vi "excelReport1.vi"(6 "device":string, 7 "Customer":string, 8 "Shift":string(combo), 9 "End Date":string="2014/9/24", 11 "From Date":string="2014/9/20") -> ()   [LabVIEW 2012]
uses:
  <vilib>/Utility/NIReport.llb/Generate Report Object Reference.ctl
  <vilib>/Utility/NIReport.llb/NI_report.lvclass
  <vilib>/addons/database/Auxilliary.llb/DB Tools Cursor Type.ctl
  <vilib>/addons/database/Connection.llb/DB Tools Open Connec (Path).vi
  <vilib>/addons/database/Connection.llb/Conn Execute.vi
  <vilib>/addons/database/Recordset.llb/Rec Fetch Recordset Data (R).vi
  <vilib>/addons/database/Recordset.llb/Rec Destroy - Connection.vi
  <vilib>/Utility/NIReport.llb/Append Text Table to Report (wrap).vi
  <vilib>/addons/database/_DB Variant To Data/Database Variant To Data.xnode
  <vilib>/addons/database/NI_Database_API.lvlib
  <vilib>/Utility/NIReport.llb/Excel/NI_Excel.lvclass
  <vilib>/addons/_office/NI_ReportGenerationToolkit.lvlib
panel:
  out "Row Headers":string[](array[string])
  out "error out":errorcluster
  out "report out":T1
  in  "Report Template":path=path "c:/m100/data/AT.xls"
  in  "Running":string[][](table)
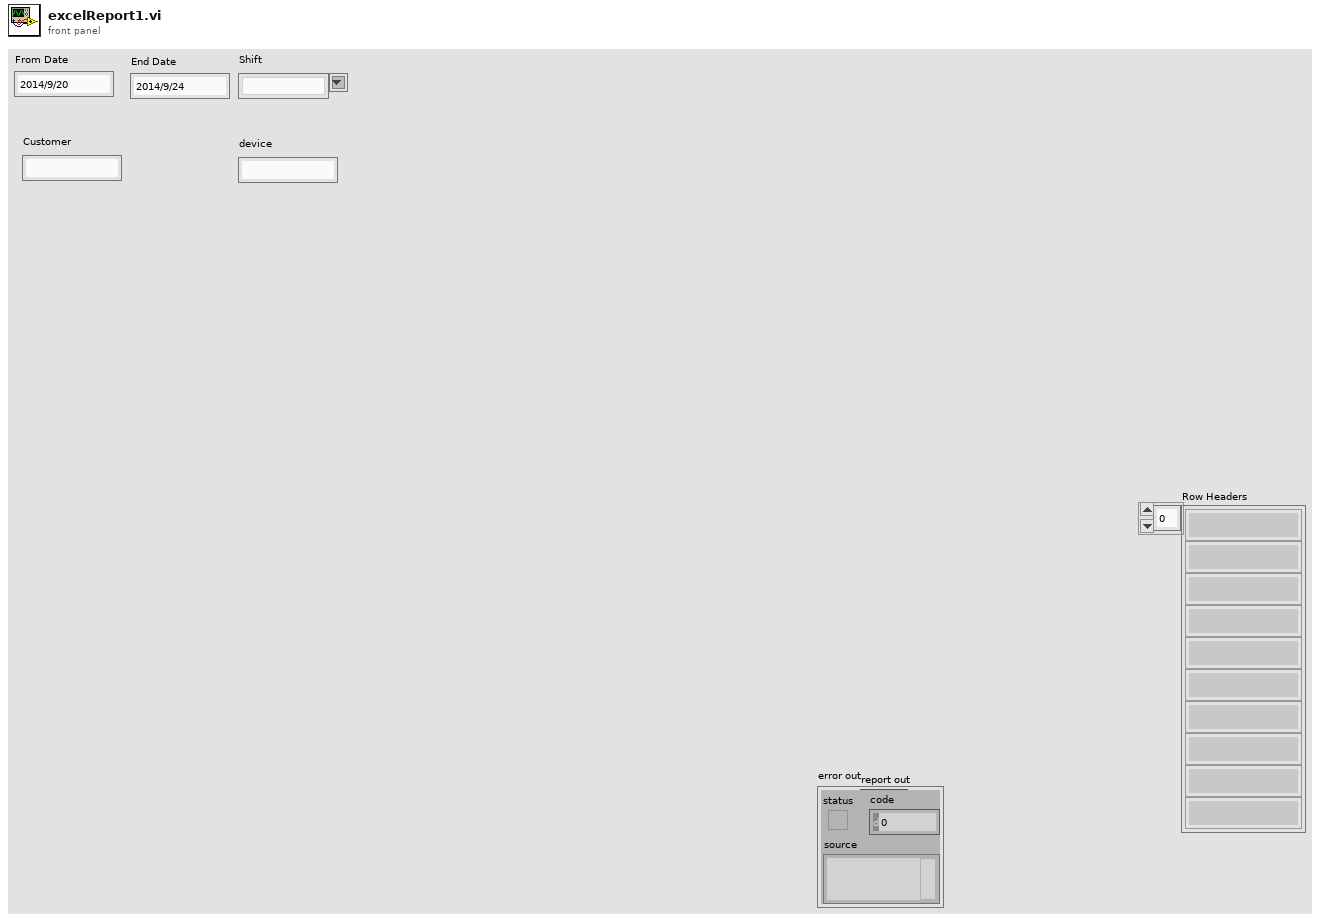
[diagram p1: front panel]
types:
  T1 = typedef "Generate Report Object Reference.ctl" = refnum<class "NI_report.lvclass">
  T2 = typedef "NI_Database_API.lvlib/DB Tools Cursor Type.ctl" = enum16{"forward-only", "keyset", "dynamic", "static"}
  T3 = typedef "NI_Database_API.lvlib/Conn ObjectReference.ctl" = refnum<k1>
  T4 = typedef "NI_Database_API.lvlib/Rec ObjectReference.ctl" = refnum<k1>
  T5 = enum16{"Standard Report", "HTML", "Word", "Excel"}
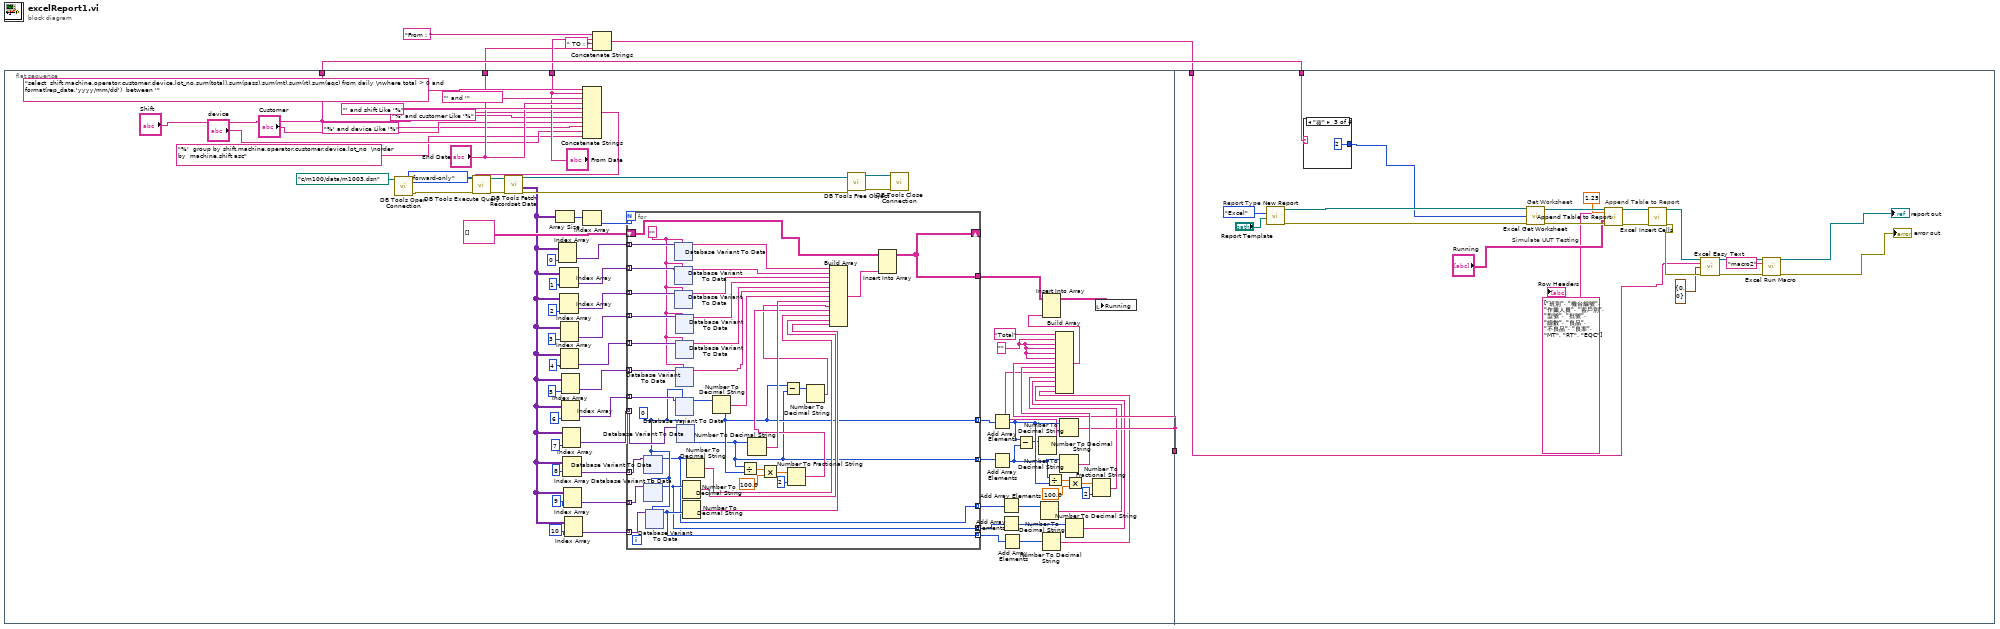
[diagram p0: block diagram]
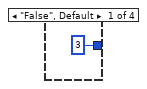
[diagram p2: hidden frame]
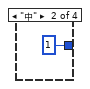
[diagram p3: hidden frame]
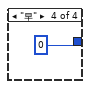
[diagram p4: hidden frame]
diagram:
  n1 = flat-sequence {
    tunnel: [w42] -> w7
    tunnel: ["Shift"] -> w6
    tunnel: ["From Date"] -> w4
    tunnel: ["End Date"] -> w2
    tunnel: w7 -> [_]
    tunnel: w6 -> [w481]
    tunnel: w1 -> [w479]
    frame #0 {
      w57 = "" ("element")
      n2 = call-poly <vilib>:"DB Tools Open Connection.vi"("connection information"=path "c:/m100/data/m1003.dsn") -> ("error out"=w47:errorcluster, "connection reference"=w48:T3)  [unwired: 7 in]
      n3 = Concatenate Strings("select  shift,machine,operator,customer,device,lot_no,sum(total),sum(pass),sum(mt),sum(rt),sum(eqc) from daily \nwhere total > 0 and  format(rep_date,'yyyy/mm/dd')  between '" ("string"), "From Date", "' and '" ("string"), "End Date", "' and shift Like '%" ("string"), "Shift", "%' and customer Like '%" ("string"), "Customer", "%' and device Like '%" ("string"), "device", "%'  group by shift,machine,operator,customer,device,lot_no  \norder by  machine,shift asc" ("string")) -> (w44:string)
      n4 = call-poly <vilib>:"DB Tools Execute Query.vi"("error in (no error)"=w47, "cursor type"=DB_Tools_Cursor_Type."forward-only", "SQL query"=w44, "connection reference"=w48) -> ("error out"=w50:errorcluster, "recordset reference"=w49:T4)  [unwired: 4 in]
      n5 = call-poly <vilib>:"DB Tools Fetch Recordset Data.vi"("error in (no error)"=w50, "recordset reference"=w49) -> ("error out"=w46:errorcluster, "recordset data"=w8:variant[][], "recordset reference out"=w45:T4)  [unwired: 3 in]
      n6 = Array Size(array=w8) -> (size(s)=w81:i32[])
      n7 = Index Array(array=w8, index (col)=0) -> (element=w70:variant[])  [unwired: 1 in]
      n8 = Index Array(array=w8, index (col)=1) -> (element=w77:variant[])  [unwired: 1 in]
      n9 = Index Array(array=w8, index (col)=2) -> (element=w69:variant[])  [unwired: 1 in]
      n10 = Index Array(array=w8, index (col)=3) -> (element=w68:variant[])  [unwired: 1 in]
      n11 = Index Array(array=w8, index (col)=4) -> (element=w67:variant[])  [unwired: 1 in]
      n12 = Index Array(array=w8, index (col)=5) -> (element=w63:variant[])  [unwired: 1 in]
      n13 = Index Array(array=w8, index (col)=6) -> (element=w66:variant[])  [unwired: 1 in]
      n14 = Index Array(array=w8, index (col)=7) -> (element=w65:variant[])  [unwired: 1 in]
      n15 = Index Array(array=w8, index (col)=8) -> (element=w31:variant[])  [unwired: 1 in]
      n16 = Index Array(array=w8, index (col)=9) -> (element=w30:variant[])  [unwired: 1 in]
      n17 = Index Array(array=w8, index (col)=10) -> (element=w29:variant[])  [unwired: 1 in]
      n18 = Index Array(array=w81) -> (element=w80:i32)  [unwired: 1 in]
      n19 = for {
        N: w80 -> [_]
        tunnel: w77 -> [w119] mode=indexing
        tunnel: w65 -> [w121] mode=indexing
        shift-right: [w98] -> _
        shift-left: string[][] [] -> [w105]
        tunnel: w70 -> [w120] mode=indexing
        tunnel: w69 -> [w118] mode=indexing
        tunnel: w68 -> [w117] mode=indexing
        tunnel: w67 -> [w116] mode=indexing
        tunnel: w66 -> [w115] mode=indexing
        tunnel: w63 -> [w112] mode=indexing
        tunnel: [w86] -> w18 mode=indexing
        tunnel: [w85] -> w61 mode=indexing
        tunnel: [w98] -> w40
        tunnel: w31 -> [w97] mode=indexing
        tunnel: w30 -> [w96] mode=indexing
        tunnel: w29 -> [w95] mode=indexing
        tunnel: [w93] -> w26 mode=indexing
        tunnel: [w92] -> w27 mode=indexing
        tunnel: [w91] -> w28 mode=indexing
        w94 = 0
        w111 = ""
        n20 = xnode "Database Variant To Data"("database variant"=w97, "type"=w94) -> ("data"=w91:i32)  [unwired: 1 in, 1 out]
        n21 = xnode "Database Variant To Data"("database variant"=w96, "type"=w94) -> ("data"=w92:i32)  [unwired: 1 in, 1 out]
        n22 = xnode "Database Variant To Data"("database variant"=w95, "type"=w94) -> ("data"=w93:i32)  [unwired: 1 in, 1 out]
        n23 = xnode "Database Variant To Data"("database variant"=w120, "type"=w111) -> ("data"=w104:string)  [unwired: 1 in, 1 out]
        n24 = xnode "Database Variant To Data"("database variant"=w119, "type"=w111) -> ("data"=w103:string)  [unwired: 1 in, 1 out]
        n25 = xnode "Database Variant To Data"("database variant"=w118, "type"=w111) -> ("data"=w99:string)  [unwired: 1 in, 1 out]
        n26 = xnode "Database Variant To Data"("database variant"=w117, "type"=w111) -> ("data"=w102:string)  [unwired: 1 in, 1 out]
        n27 = xnode "Database Variant To Data"("database variant"=w116, "type"=w111) -> ("data"=w101:string)  [unwired: 1 in, 1 out]
        n28 = xnode "Database Variant To Data"("database variant"=w115, "type"=w94) -> ("data"=w86:i32)  [unwired: 1 in, 1 out]
        n29 = xnode "Database Variant To Data"("database variant"=w112, "type"=w111) -> ("data"=w100:string)  [unwired: 1 in, 1 out]
        n30 = xnode "Database Variant To Data"("database variant"=w121, "type"=w94) -> ("data"=w85:i32)  [unwired: 1 in, 1 out]
        n31 = Number To Decimal String(number=w92) -> (decimal integer string=w89:string)  [unwired: 1 in]
        n32 = Number To Decimal String(number=w93) -> (decimal integer string=w90:string)  [unwired: 1 in]
        n33 = Number To Decimal String(number=w91) -> (decimal integer string=w88:string)  [unwired: 1 in]
        n34 = Number To Decimal String(number=w86) -> (decimal integer string=w109:string)  [unwired: 1 in]
        n35 = Divide(x=w85, y=w86) -> (x/y=w113:dbl)
        n36 = Number To Decimal String(number=w85) -> (decimal integer string=w110:string)  [unwired: 1 in]
        n37 = Multiply(x=w113, y=100.0) -> (x*y=w108:dbl)
        n38 = Subtract(x=w86, y=w85) -> (x-y=w84:i32)
        n39 = Number To Fractional String(number=w108, precision (6)=i16 2) -> (F-format string=w87:string)  [unwired: 2 in]
        n40 = Number To Decimal String(number=w84) -> (decimal integer string=w83:string)  [unwired: 1 in]
        n41 = Build Array(w104, w103, w99, w102, w101, w100, w109, w110, w83, w87, w88, w89, w90) -> (w106:string[])
        n42 = Insert Into Array(array=w105, new element=w106) -> (w98:string[][])  [unwired: 2 in]
      }
      n43 = call-poly <vilib>:"DB Tools Free Object.vi"("error in (no error)"=w46, "recordset reference"=w45) -> ("error out"=w51:errorcluster, "connection reference"=w52:T3)  [unwired: 8 in]
      n44 = call <vilib>:"DB Tools Close Connection.vi"("error in (no error)"=w51, "connection reference"=w52) -> ()  [unwired: 5 in, 1 out]
      n45 = Add Array Elements(numeric array=w61) -> (sum=w16:i32)
      n46 = Add Array Elements(numeric array=w18) -> (sum=w17:i32)
      n47 = Add Array Elements(numeric array=w28) -> (sum=w25:i32)
      n48 = Add Array Elements(numeric array=w27) -> (sum=w24:i32)
      n49 = Add Array Elements(numeric array=w26) -> (sum=w23:i32)
      n50 = Subtract(x=w17, y=w16) -> (x-y=w15:i32)
      n51 = Number To Decimal String(number=w15) -> (decimal integer string=w14:string)  [unwired: 1 in]
      n52 = Number To Decimal String(number=w25) -> (decimal integer string=w20:string)  [unwired: 1 in]
      n53 = Number To Decimal String(number=w23) -> (decimal integer string=w22:string)  [unwired: 1 in]
      n54 = Divide(x=w16, y=w17) -> (x/y=w55:dbl)
      n55 = Number To Decimal String(number=w17) -> (decimal integer string=w42:string)  [unwired: 1 in]
      n56 = Number To Decimal String(number=w16) -> (decimal integer string=w59:string)  [unwired: 1 in]
      n57 = Number To Decimal String(number=w24) -> (decimal integer string=w21:string)  [unwired: 1 in]
      n58 = Multiply(x=w55, y=100.0) -> (x*y=w54:dbl)
      n59 = Number To Fractional String(number=w54, precision (6)=i16 2) -> (F-format string=w19:string)  [unwired: 2 in]
      n60 = Build Array("Total", w57, w57, w57, w57, w57, w42, w59, w14, w19, w20, w21, w22) -> (w58:string[])
      n61 = Insert Into Array(array=w40, new element=w58) -> (w41:string[][])  [unwired: 2 in]
      n62 = local write "Running"(w41) -> ()
    }
    frame #1 {
      w489 = string[] ["班別", "機台編號", "作業人員", "客戶別", "型號", "批號", "總數", "良品", "不良品", "良率", "MT", "RT", "EQC"] ("row headers")
      w495 = T5."Excel"  # Report Type
      # "Simulate UUT Testing"
      # "Append Table to Report"
      # "Get Worksheet"
      n63 = call <vilib>:"New Report.vi"("report type"=w495, "template (empty)"="Report Template") -> ("report out"=w483:refnum<class "NI_report.lvclass">, "error out"=w482:errorcluster)  [unwired: 12 in]
      n64 = case shown="\"夜\"" w481 {
        tunnel: [3 1 2 0] -> w480
        frame "False", Default {
        }
        frame "中" {
        }
        frame "夜" {
        }
        frame "早" {
        }
      }
      n65 = call <vilib>:"Excel Get Worksheet.vi"("report in"=w483, "worksheet index (0)"=w480, "error in (no error)"=w482) -> ("report out"=w493:refnum<class "NI_report.lvclass">, "error out"=w492:errorcluster)  [unwired: 11 in]
      n66 = call-poly <vilib>:"Append Table to Report.vi"("report in"=w493, "column width (1)"=1.25, "column headers"=w489, "text data"="Running", "error in (no error)"=w492) -> ("report out"=w488:refnum<class "NI_report.lvclass">, "error out"=w487:errorcluster)  [unwired: 7 in, 2 out]
      n67 = call <vilib>:"Excel Insert Cells.vi"("report in"=w488, "error in (no error)"=w487) -> ("report out"=w486:refnum<class "NI_report.lvclass">, "error out"=w485:errorcluster)  [unwired: 12 in]
      n68 = call <vilib>:"Excel Easy Text.vi"("report in"=w486, "text"=w479, "start (-1, -1)"=cluster{"row":i32, "column":i32} {"row"=0, "column"=0} ("end (-1, -1)"), "error in (no error)"=w485) -> ("report out"=w478:refnum<class "NI_report.lvclass">, "error out"=w477:errorcluster)  [unwired: 7 in, 3 out]
      n69 = call <vilib>:"Excel Run Macro.vi"("report in"=w478, "macro name"="macro2", "error in (no error)"=w477) -> ("report out"=→"report out":refnum<class "NI_report.lvclass">, "error out"=→"error out":errorcluster)  [unwired: 10 in, 1 out]
      "Row Headers" <- w489
    }
  }
  n70 = Concatenate Strings("From : " ("string"), w4, " TO : " ("string"), w2) -> (w1:string)
